vi "Normalize Path.vi"(3 "Path String":string) -> (1 "Path":path)   [LabVIEW 2020, in "Volatus.lvlib"]
uses:
  Volatus.lvlib
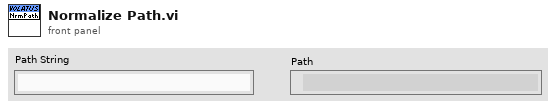
[diagram p1: front panel]
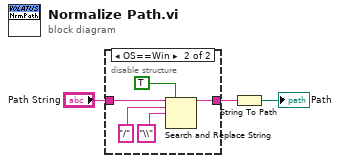
[diagram p0: block diagram]
diagram:
  n1 = disable-structure shown="OS==Win" {
    disable-tunnel: "Path String" -> [w4 w9]
    disable-tunnel: [w4 w5] -> w2
    frame condition #0 {
    }
    frame condition #1 (active) {
      n2 = Search and Replace String(replace all?=TRUE ("replace all? (F)"), input string=w9, search string="/", replace string="\\") -> (result string=w5:string)  [unwired: 4 in, 3 out]
    }
  }
  n3 = String To Path(string=w2) -> (path=→"Path":path)
